vi "总氮总磷质控流程.vi"(0 "队列输入TP":refnum<queue>, 1 "队列输入TN":refnum<queue>, 5 "总氮量程切换":enum32{"H", "L", "AUTO"}(ring)=enum."AUTO", 7 "总磷量程切换":enum32{"H", "L", "AUTO"}(ring)=enum."AUTO", 9 "总磷":bool, 11 "总氮":bool) -> (4 "布尔":bool, 6 "总磷中断报警":bool, 8 "总氮中断报警":bool)   [LabVIEW 2016, in "质控单元.lvlib"]
panel:
  out "总磷":bool
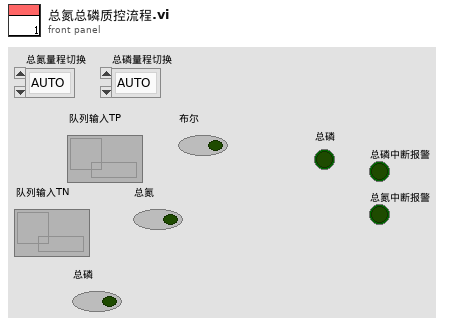
[diagram p1: front panel]
types:
  T1 = enum16{"待机", "启动氨氮水样", "氨氮测量中", "启动氨氮加标", "启动氨氮加标回收", "氨氮加标回收测量中", "启动总氮水样", "总氮测量中", "启动总氮加标", "启动总氮加标回收", "总氮加标回收测量中", "启动总磷水样", "总磷水样测量中", "启动总磷加标", "启动总磷加标回收", "总磷加标回收测量中", "结束"}
  T2 = cluster{"时间标识":timestamp, "设备":string, "日志信息":string}
  T3 = cluster{"站号":u16, "量程切换":enum32{"H", "L", "AUTO"}, "控制命令":enum16{"启动测量", "标样核查", "零点核查", "跨度核查", "空白测试", "平行样测试", "加标回收", "空白校准", "标样校准", "初始化（清洗）", "停止测试", "仪器重启", "校时", "模式设置", "测量间隔设置"}, "模式设置":enum16{"待机", "连续模式", "周期模式", "定点模式", "受控模式", "手动模式"}, "测量间隔":u16}
  T4 = cluster{"系统时间":timestamp, "工作状态":enum16{"空闲", "水样测试", "标样核查", "零点核查", "跨度核查", "空白测试", "平行样测试", "加标回收", "空白校准", "标样校准", "初始化（清洗）"}, "测量模式":enum16{"待机", "连续模式", "周期模式", "定点模式", "受控模式", "手动模式"}, "告警代码":enum16{"无告警", "缺试剂告警", "缺水样告警", "缺蒸馏水告警", "缺标液告警", "仪表漏液告警", "标定异常告警", "超量程告警", "加热异常", "低试剂预警", "超上限告警", "超下限告警", "仪表内部其他异常", "滴定异常告警", "电极异常告警", "量程切换告警", "参数设置告警", "PH电极电位异常", "电导率电极异常", "浊度光度异常", "溶解氧电极异常", "溶解氧光强异常", "温度异常告警", "PH异常告警", "溶解氧异常告警", "电导率异常告警", "浊度异常告警", "叶绿素异常告警", "藻密度异常告警", "蓝绿藻异常告警", "ORP异常告警", "氨氮异常告警", "清洁刷异常告警", "SD卡异常告警", "蓝牙异常告警", "Wifi异常告警", "流程异常告警"}, "故障代码":enum16{"无故障", "电机故障", "温度故障", "通讯故障", "滴定故障"}, "日志代码":u16, "软件版本":u16, "F0":sgl, "F1":sgl, "F2":sgl, "F3":sgl, "T":sgl, "H":sgl, "id":u16, "flowid":u16, "量程":u16, "总磷控温温度1":sgl, "营养盐控温温度2":sgl, "ADC":sgl}
  T5 = enum16{"空闲", "水样测试", "标样核查", "零点核查", "跨度核查", "空白测试", "平行样测试", "加标回收", "空白校准", "标样校准", "初始化（清洗）"}
  T6 = cluster{"因子编码":u32, "单位":u16, "标样参考值":sgl, "水样数据时间":timestamp, "水样实测值":sgl, "水样数据标识":string, "标样数据时间":timestamp, "标样实测值":sgl, "标样数据标识":string, "空白数据时间":timestamp, "空白实测值":sgl, "空白数据标识":string, "零点核查数据时间":timestamp, "零点核查实测值":sgl, "零点核查数据标识":string, "跨度核查数据时间":timestamp, "跨度核查实测值":sgl, "跨度核查数据标识":string, "加标回收数据时间":timestamp, "加标回收实测值":sgl, "加标回收数据标识":string, "平行样数据时间":timestamp, "平行样实测值":sgl, "平行样数据标识":string, "F0":sgl, "F1":sgl, "F2":sgl, "F3":sgl, "F4":sgl, "F5":sgl, "F6":sgl, "F7":sgl, "温度":sgl, "湿度":sgl, "X值":sgl}
  T7 = cluster{"量程":dbl, "检出限":dbl, "加标前水样浓度":dbl, "加标后水样浓度":dbl, "加标水杯定容体积":dbl, "加标母液浓度":dbl, "加标体积":dbl, "加标回收率":dbl}
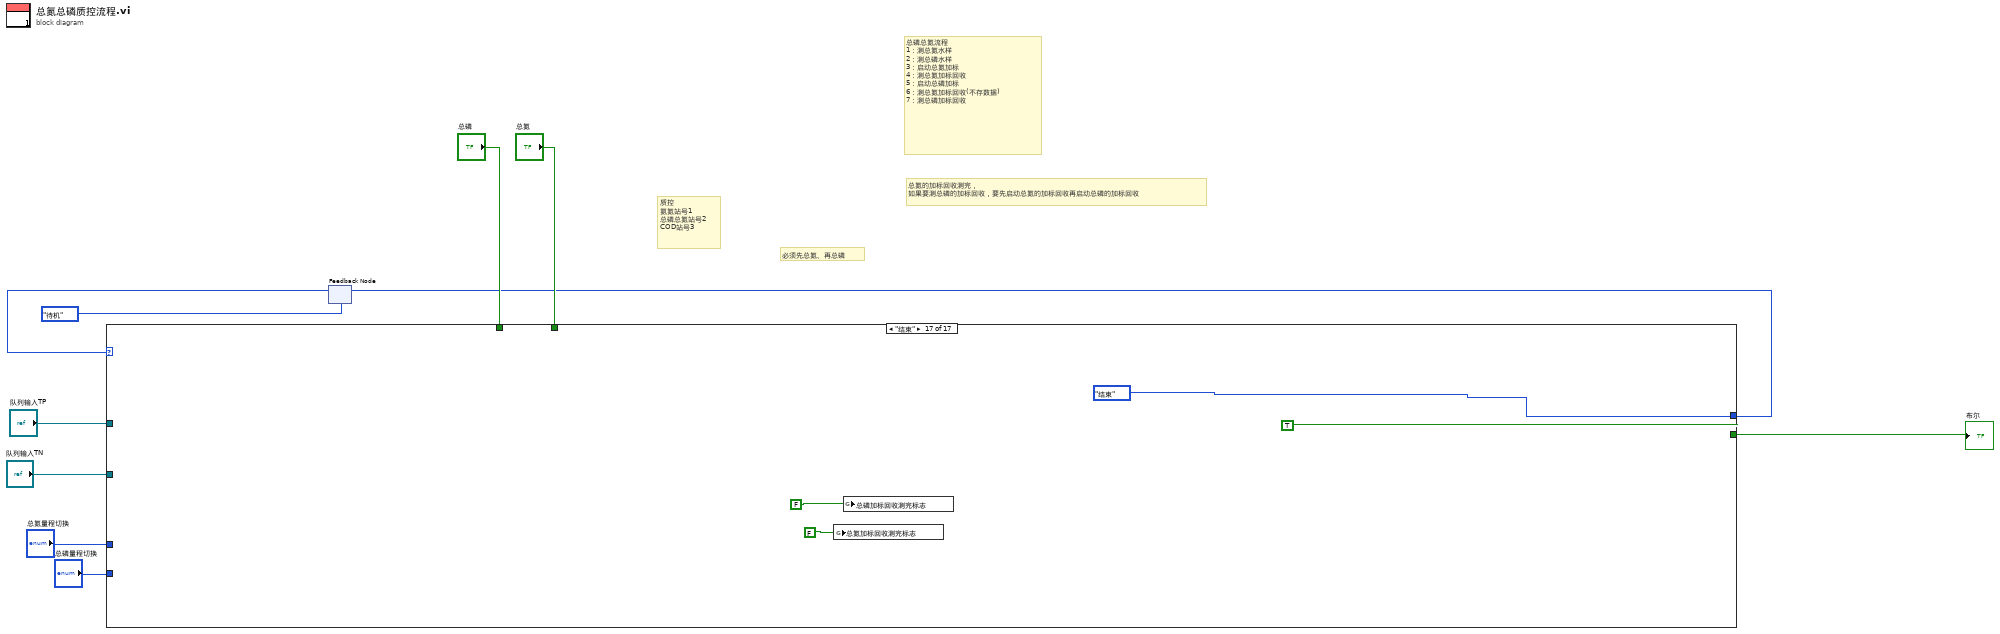
[diagram p0: block diagram]
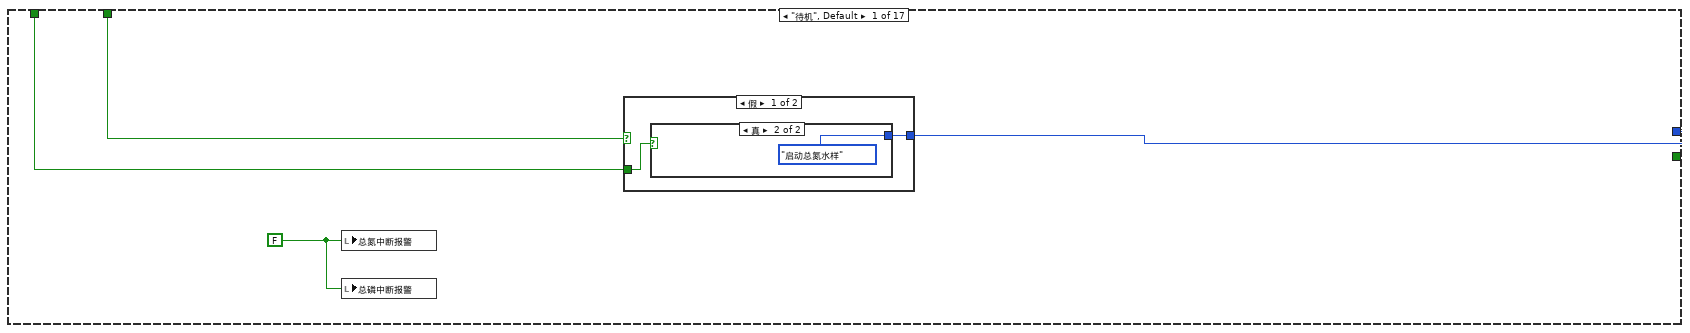
[diagram p2: hidden frame]
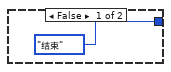
[diagram p3: hidden frame]
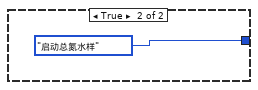
[diagram p4: hidden frame]
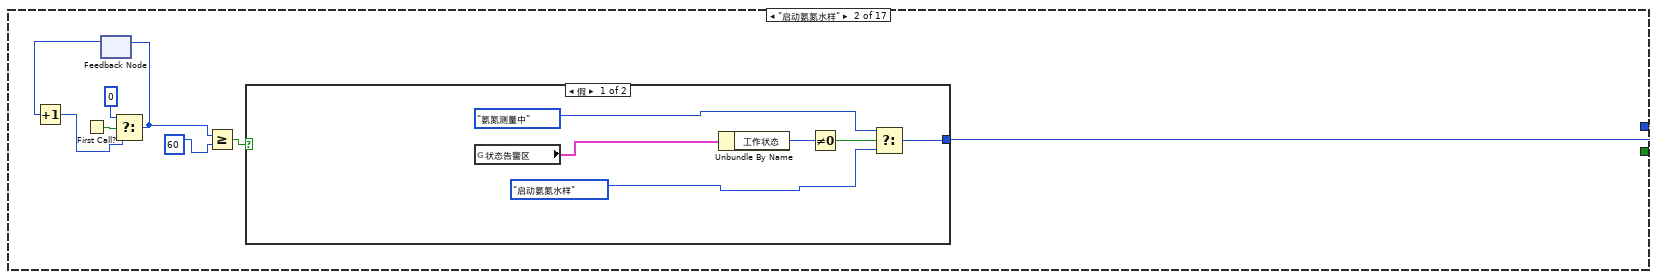
[diagram p5: hidden frame]
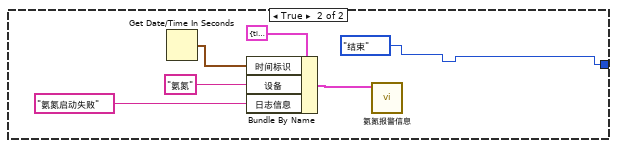
[diagram p6: hidden frame]
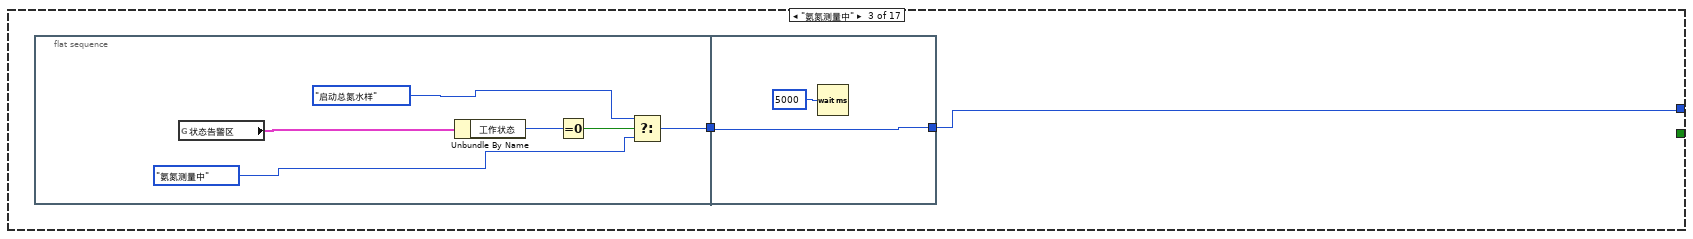
[diagram p7: hidden frame]
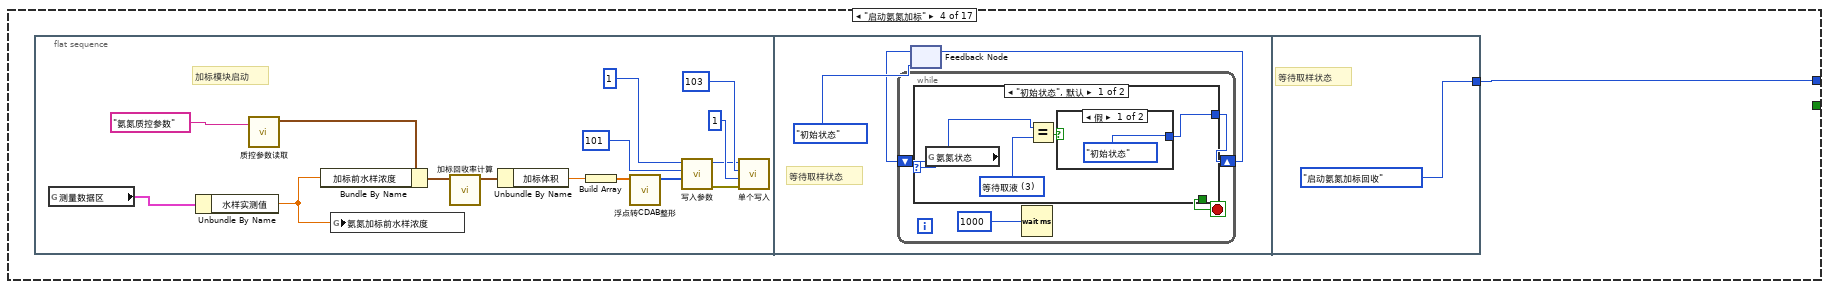
[diagram p8: hidden frame]
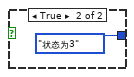
[diagram p9: hidden frame]
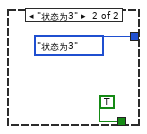
[diagram p10: hidden frame]
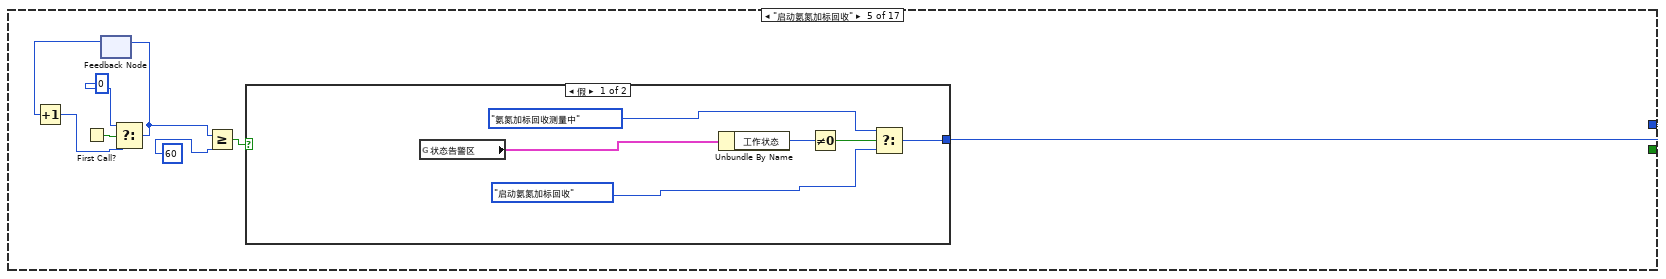
[diagram p11: hidden frame]
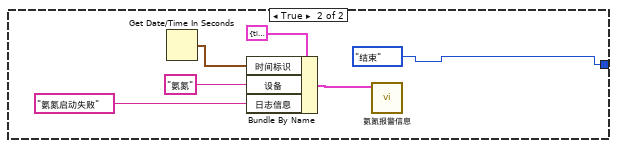
[diagram p12: hidden frame]
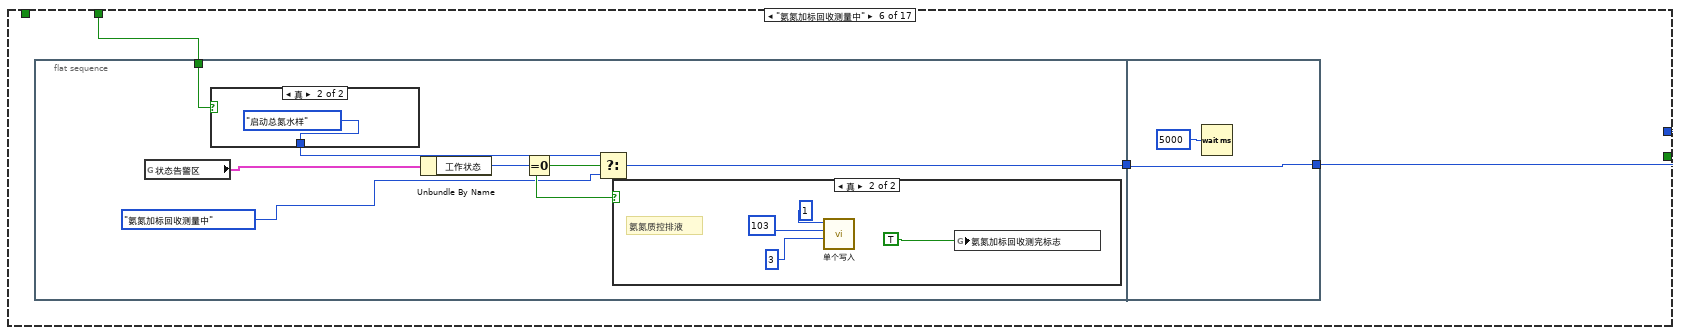
[diagram p13: hidden frame]
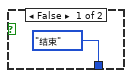
[diagram p14: hidden frame]
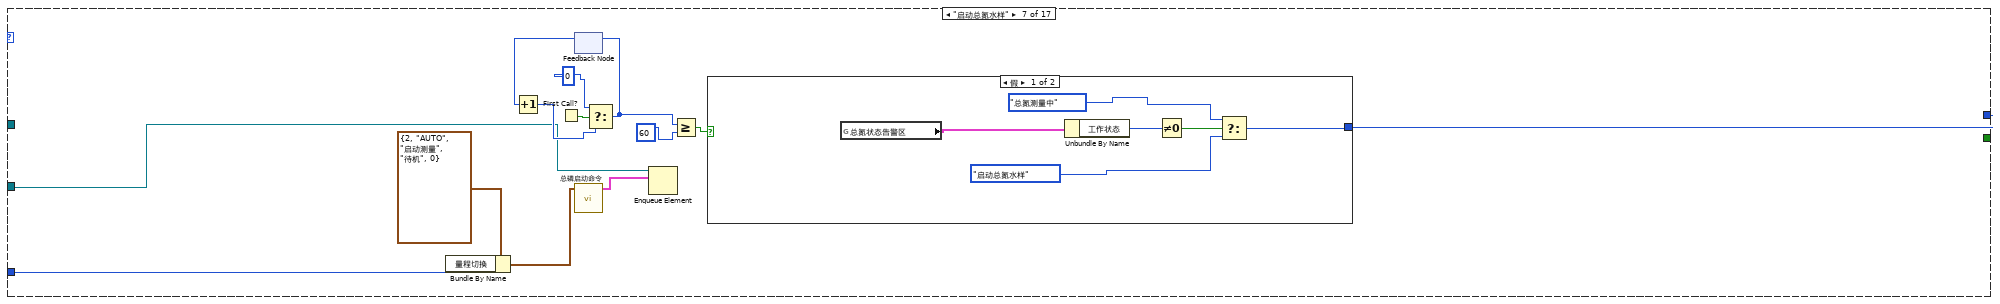
[diagram p16: hidden frame]
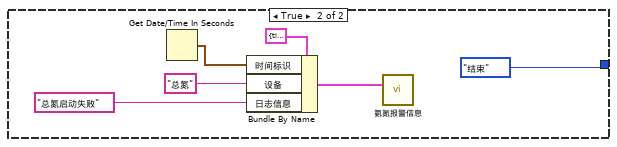
[diagram p17: hidden frame]
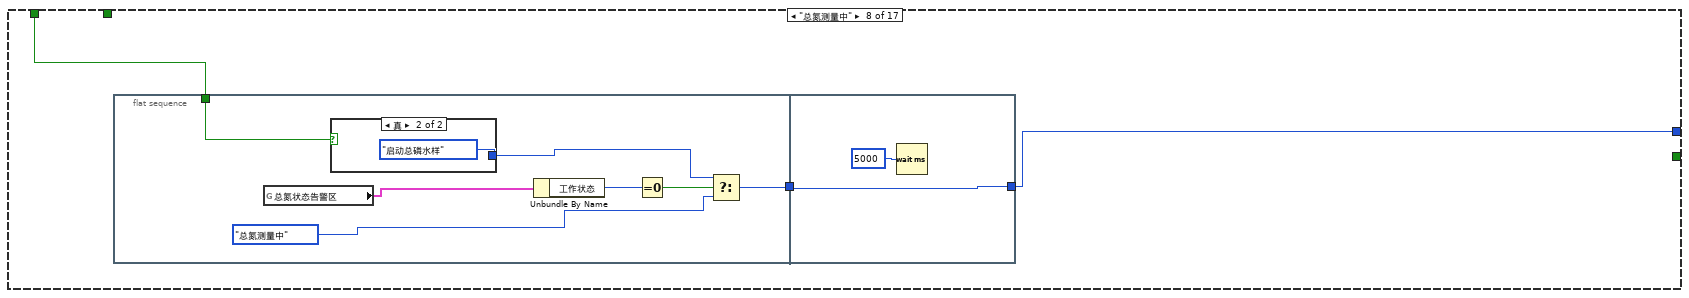
[diagram p18: hidden frame]
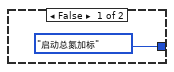
[diagram p19: hidden frame]
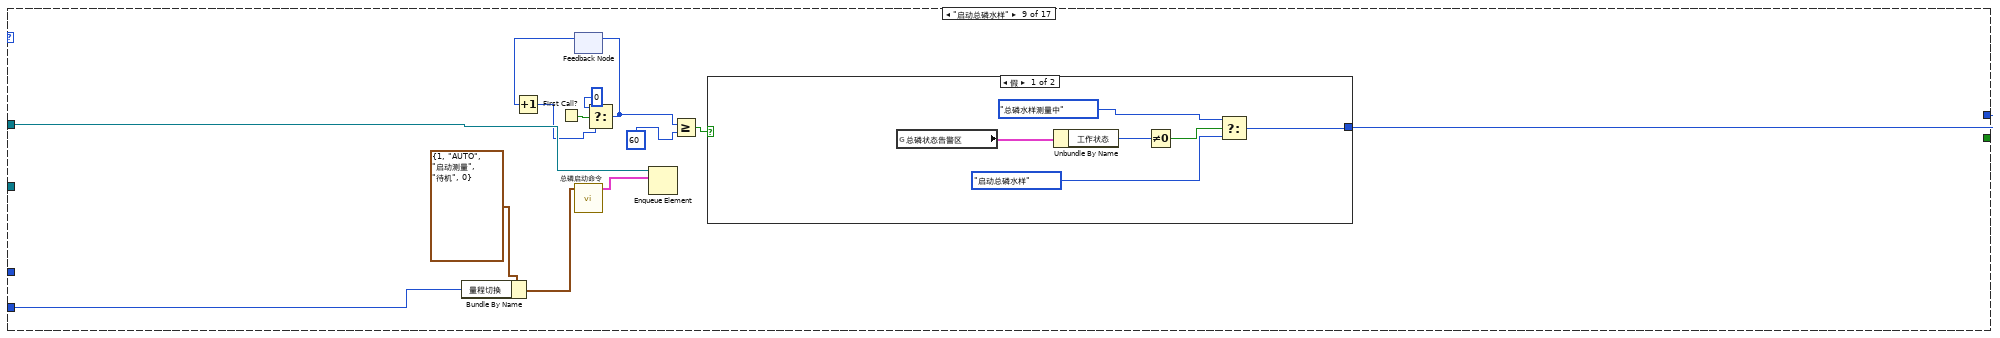
[diagram p20: hidden frame]
diagram:
  # "总磷总氮流程\n1：测总氮水样\n2：测总磷水样\n3：启动总氮加标\n4：测总氮加标回收\n5：启动总磷加标\n6：测总氮加标回收(不存数据)\n7：测总磷加标回收"
  # "总氮的加标回收测完，\n如果要测总磷的加标回收，要先启动总氮的加标回收再启动总磷的加标回收"
  # "质控\n氨氮站号1   \n总磷总氮站号2\nCOD站号3"
  # "必须先总氮、再总磷"
  n1 = feedback #1(T1."待机") -> (w6:T1)
  n2 = case shown="\"结束\"" w6 {
    tunnel: [w14 w27 w41 w50 w81 w101 w131 w145 w169 w185 w197 w238 w260 w288 w331 w353 T1."结束"] -> w4
    tunnel: "队列输入TP" -> [_ _ _ _ _ _ _ _ w170 _ _ _ _ _ w332 _ _]
    tunnel: [_ _ _ _ _ _ _ _ _ _ _ _ _ _ _ _ TRUE] -> w9
    tunnel: "总磷" -> [w13 _ _ _ _ _ _ w144 _ _ _ _ w261 _ _ _ _]
    tunnel: "总氮" -> [w12 _ _ _ _ w102 _ _ _ w183 _ _ w259 _ _ _ _]
    tunnel: "总氮量程切换" -> [_ _ _ _ _ _ w120 _ _ _ _ w235 _ _ _ _ _]
    tunnel: "总磷量程切换" -> [_ _ _ _ _ _ _ _ w158 _ _ _ _ _ w327 _ _]
    tunnel: "队列输入TN" -> [_ _ _ _ _ _ w119 _ _ _ _ w234 _ _ _ _ _]
    frame "待机", Default {
      w11 = FALSE ("总氮中断报警")
      n3 = local write "总氮中断报警"(w11) -> ()
      n4 = local write "总磷中断报警"(w11) -> ()
      n5 = case shown="假" w12 {
        tunnel: w13 -> [w15 _]
        tunnel: [w16 T1."启动总氮水样"] -> w14
        frame False {
          n6 = case shown="真" w15 {
            tunnel: [T1."结束" T1."启动总氮水样"] -> w16
            frame False {
            }
            frame True {
            }
          }
        }
        frame True {
        }
      }
    }
    frame "启动氨氮水样" {
      n7 = First Call?() -> (First Call?: T/F=w25:bool)
      n8 = feedback #2() -> (w24:i32)  [unwired: 1 in]
      n9 = Increment(x=w24) -> (x+1=w23:i32)
      n10 = Select(t=0, s=w25, f=w23) -> (s? t:f=w22:i32)
      n11 = feedback-in #2(w22) -> ()
      n12 = Greater Or Equal?(x=w22, y=60) -> (x >= y?=w20:bool)
      n13 = case shown="假" w20 {
        tunnel: [w31 T1."结束"] -> w27
        frame False {
          n14 = global read "VAR氨氮全局变量.vi" "状态告警区"() -> (w28:T4)
          n15 = Unbundle By Name(w28) -> ("工作状态"=w33:T5)
          n16 = Not Equal To 0?(x=w33) -> (x != 0?=w32:bool)
          n17 = Select(t=T1."氨氮测量中", s=w32, f=T1."启动氨氮水样") -> (s? t:f=w31:T1)
        }
        frame True {
          n18 = Get Date/Time In Seconds() -> (seconds since 1Jan1904=w39:timestamp)
          n19 = Bundle By Name(cluster=T2 {"时间标识"=timestamp(0 s since 1904-01-01), "设备"="", "日志信息"=""} ("data in"), "时间标识"=w39, "设备"="氨氮", "日志信息"="氨氮启动失败") -> (w35:T2)
          n20 = call "氨氮报警信息.vi"("data in"=w35) -> ()  [unwired: 10 in, 1 out]
        }
      }
    }
    frame "氨氮测量中" {
      n21 = flat-sequence {
        tunnel: [w46] -> w40
        tunnel: [w49] -> w41
        tunnel: w40 -> [w49]
        frame #0 {
          n22 = global read "VAR氨氮全局变量.vi" "状态告警区"() -> (w42:T4)
          n23 = Unbundle By Name(w42) -> ("工作状态"=w47:T5)
          n24 = Equal To 0?(x=w47) -> (x = 0?=w45:bool)
          n25 = Select(t=T1."启动总氮水样", s=w45, f=T1."氨氮测量中") -> (s? t:f=w46:T1)
        }
        frame #1 {
          n26 = Wait (ms)(milliseconds to wait=u32 5000 ("等待时间（毫秒）")) -> ()  [unwired: 1 out]
        }
      }
    }
    frame "启动氨氮加标" {
      n27 = flat-sequence {
        tunnel: [T1."启动氨氮加标回收"] -> w50
        frame #0 {
          w54 = u16 1 ("value")
          # "加标模块启动"
          n28 = global read "VAR氨氮全局变量.vi" "测量数据区"() -> (w51:T6)
          n29 = Unbundle By Name(w51) -> ("水样实测值"=w52:sgl)
          n30 = call "质控参数读取.vi"("section"="氨氮质控参数") -> ("参数"=w62:T7)  [unwired: 9 in, 1 out]
          n31 = Bundle By Name(cluster=w62, "加标前水样浓度"=w52) -> (w63:T7)
          n32 = global write "水样浓度全局.vi" "氨氮加标前水样浓度"(w52) -> ()
          n33 = call "加标回收率计算.vi"("参数"=w63) -> ("参数 out"=w61:T7)  [unwired: 10 in]
          n34 = Unbundle By Name(w61) -> ("加标体积"=w53:dbl)
          n35 = Build Array(w53) -> (w60:dbl[])
          n36 = call "浮点转CDAB整形.vi"("浮点数"=w60) -> ("CDAB整形输出"=w55:u16[])  [unwired: 10 in]
          n37 = call "写入参数.vi"("values"=w55, "starting address"=u16 101, "Slave ID"=w54) -> ("error out"=w59:errorcluster)  [unwired: 8 in]
          n38 = call "单个写入.vi"("Error in"=w59, "value"=u16 1, "address"=u16 103, "Slave ID"=w54) -> ()  [unwired: 7 in, 1 out]
        }
        frame #1 {
          # "等待取样状态"
          n39 = feedback #3(enum16{"初始状态", "状态为3"}."初始状态") -> (w66:enum16{"初始状态", "状态为3"})
          n40 = while {
            shift-right: [w70] -> w65
            shift-left: w66 -> [w71]
            stop <- w69 stop-if-true
            n41 = case shown="\"初始状态\", 默认" w71 {
              tunnel: [w73 enum16{"初始状态", "状态为3"}."状态为3"] -> w70
              tunnel: [_ TRUE] -> w69
              frame "初始状态", Default {
                w72 = u16 3 items=["待机", "润洗", "进样", "等待取液", "排液"] ("氨氮状态")
                n42 = global read "氨氮加标回收状态全局变量.vi" "氨氮状态"() -> (w75:u16)
                n43 = Equal?(x=w75, y=w72) -> (x = y?=w74:bool)
                n44 = case shown="假" w74 {
                  tunnel: [enum16{"初始状态", "状态为3"}."初始状态" enum16{"初始状态", "状态为3"}."状态为3"] -> w73
                  frame False {
                  }
                  frame True {
                  }
                }
              }
              frame "状态为3" {
              }
            }
            n45 = Wait (ms)(milliseconds to wait=u32 1000 ("等待时间（毫秒）")) -> ()  [unwired: 1 out]
          }
          n46 = feedback-in #3(w65) -> ()
        }
        frame #2 {
          # "等待取样状态"
        }
      }
    }
    frame "启动氨氮加标回收" {
      n47 = First Call?() -> (First Call?: T/F=w87:bool)
      n48 = feedback #4() -> (w86:i32)  [unwired: 1 in]
      n49 = Increment(x=w86) -> (x+1=w85:i32)
      n50 = Select(t=0, s=w87, f=w85) -> (s? t:f=w84:i32)
      n51 = feedback-in #4(w84) -> ()
      n52 = Greater Or Equal?(x=w84, y=60) -> (x >= y?=w82:bool)
      n53 = case shown="假" w82 {
        tunnel: [w92 T1."结束"] -> w81
        frame False {
          n54 = global read "VAR氨氮全局变量.vi" "状态告警区"() -> (w89:T4)
          n55 = Unbundle By Name(w89) -> ("工作状态"=w94:T5)
          n56 = Not Equal To 0?(x=w94) -> (x != 0?=w93:bool)
          n57 = Select(t=T1."氨氮加标回收测量中", s=w93, f=T1."启动氨氮加标回收") -> (s? t:f=w92:T1)
        }
        frame True {
          n58 = Get Date/Time In Seconds() -> (seconds since 1Jan1904=w100:timestamp)
          n59 = Bundle By Name(cluster=T2 {"时间标识"=timestamp(0 s since 1904-01-01), "设备"="", "日志信息"=""} ("data in"), "时间标识"=w100, "设备"="氨氮", "日志信息"="氨氮启动失败") -> (w96:T2)
          n60 = call "氨氮报警信息.vi"("data in"=w96) -> ()  [unwired: 10 in, 1 out]
        }
      }
    }
    frame "氨氮加标回收测量中" {
      n61 = flat-sequence {
        tunnel: [w109] -> w103
        tunnel: w102 -> [w106]
        tunnel: [w118] -> w101
        tunnel: w103 -> [w118]
        frame #0 {
          n62 = global read "VAR氨氮全局变量.vi" "状态告警区"() -> (w104:T4)
          n63 = case shown="真" w106 {
            tunnel: [T1."结束" T1."启动总氮水样"] -> w108
            frame False {
            }
            frame True {
            }
          }
          n64 = Unbundle By Name(w104) -> ("工作状态"=w110:T5)
          n65 = Equal To 0?(x=w110) -> (x = 0?=w107:bool)
          n66 = Select(t=w108, s=w107, f=T1."氨氮加标回收测量中") -> (s? t:f=w109:T1)
          n67 = case shown="真" w107 {
            frame False {
            }
            frame True {
              # "氨氮质控排液"
              n68 = call "单个写入.vi"("value"=u16 3, "address"=u16 103, "Slave ID"=u8 1) -> ()  [unwired: 8 in, 1 out]
              n69 = global write "质控测完标志全局 1.vi" "氨氮加标回收测完标志"(TRUE) -> ()
            }
          }
        }
        frame #1 {
          n70 = Wait (ms)(milliseconds to wait=u32 5000 ("等待时间（毫秒）")) -> ()  [unwired: 1 out]
        }
      }
    }
    frame "启动总氮水样" {
      n71 = Bundle By Name(cluster=T3 {"站号"=2, "量程切换"=enum."AUTO", "控制命令"=enum."启动测量", "模式设置"=enum."待机", "测量间隔"=0} ("参数"), "量程切换"=w120) -> (w121:T3)
      n72 = First Call?() -> (First Call?: T/F=w129:bool)
      n73 = feedback #5() -> (w128:i32)  [unwired: 1 in]
      n74 = Increment(x=w128) -> (x+1=w127:i32)
      n75 = call "总磷启动命令.vi"("参数"=w121) -> ("启动命令"=w123:cluster{"命令":string, "data":variant})  [unwired: 10 in]
      n76 = Select(t=0, s=w129, f=w127) -> (s? t:f=w126:i32)
      n77 = feedback-in #5(w126) -> ()
      n78 = Enqueue Element(queue=w119, element=w123) -> ()  [unwired: 2 in, 3 out]
      n79 = Greater Or Equal?(x=w126, y=60) -> (x >= y?=w124:bool)
      n80 = case shown="假" w124 {
        tunnel: [w135 T1."结束"] -> w131
        frame False {
          n81 = global read "VAR总氮全局变量.vi" "总氮状态告警区"() -> (w132:T4)
          n82 = Unbundle By Name(w132) -> ("工作状态"=w136:T5)
          n83 = Not Equal To 0?(x=w136) -> (x != 0?=w137:bool)
          n84 = Select(t=T1."总氮测量中", s=w137, f=T1."启动总氮水样") -> (s? t:f=w135:T1)
        }
        frame True {
          n85 = Get Date/Time In Seconds() -> (seconds since 1Jan1904=w143:timestamp)
          n86 = Bundle By Name(cluster=T2 {"时间标识"=timestamp(0 s since 1904-01-01), "设备"="", "日志信息"=""} ("data in"), "时间标识"=w143, "设备"="总氮", "日志信息"="总氮启动失败") -> (w139:T2)
          n87 = call "氨氮报警信息.vi"("data in"=w139) -> ()  [unwired: 10 in, 1 out]
        }
      }
    }
    frame "总氮测量中" {
      n88 = flat-sequence {
        tunnel: [w152] -> w146
        tunnel: w144 -> [w148]
        tunnel: [w157] -> w145
        tunnel: w146 -> [w157]
        frame #0 {
          n89 = global read "VAR总氮全局变量.vi" "总氮状态告警区"() -> (w147:T4)
          n90 = case shown="真" w148 {
            tunnel: [T1."启动总氮加标" T1."启动总磷水样"] -> w150
            frame False {
            }
            frame True {
            }
          }
          n91 = Unbundle By Name(w147) -> ("工作状态"=w153:T5)
          n92 = Equal To 0?(x=w153) -> (x = 0?=w151:bool)
          n93 = Select(t=w150, s=w151, f=T1."总氮测量中") -> (s? t:f=w152:T1)
        }
        frame #1 {
          n94 = Wait (ms)(milliseconds to wait=u32 5000 ("等待时间（毫秒）")) -> ()  [unwired: 1 out]
        }
      }
    }
    frame "启动总磷水样" {
      n95 = Bundle By Name(cluster=T3 {"站号"=1, "量程切换"=enum."AUTO", "控制命令"=enum."启动测量", "模式设置"=enum."待机", "测量间隔"=0} ("参数"), "量程切换"=w158) -> (w159:T3)
      n96 = First Call?() -> (First Call?: T/F=w167:bool)
      n97 = feedback #6() -> (w166:i32)  [unwired: 1 in]
      n98 = Increment(x=w166) -> (x+1=w165:i32)
      n99 = call "总磷启动命令.vi"("参数"=w159) -> ("启动命令"=w161:cluster{"命令":string, "data":variant})  [unwired: 10 in]
      n100 = Select(t=0, s=w167, f=w165) -> (s? t:f=w164:i32)
      n101 = feedback-in #6(w164) -> ()
      n102 = Enqueue Element(queue=w170, element=w161) -> ()  [unwired: 2 in, 3 out]
      n103 = Greater Or Equal?(x=w164, y=60) -> (x >= y?=w162:bool)
      n104 = case shown="假" w162 {
        tunnel: [w173 T1."结束"] -> w169
        frame False {
          n105 = global read "VAR总磷全局变量.vi" "总磷状态告警区"() -> (w174:T4)
          n106 = Unbundle By Name(w174) -> ("工作状态"=w175:T5)
          n107 = Not Equal To 0?(x=w175) -> (x != 0?=w176:bool)
          n108 = Select(t=T1."总磷水样测量中", s=w176, f=T1."启动总磷水样") -> (s? t:f=w173:T1)
        }
        frame True {
          n109 = Get Date/Time In Seconds() -> (seconds since 1Jan1904=w182:timestamp)
          n110 = Bundle By Name(cluster=T2 {"时间标识"=timestamp(0 s since 1904-01-01), "设备"="", "日志信息"=""} ("data in"), "时间标识"=w182, "设备"="总磷", "日志信息"="总磷启动失败") -> (w178:T2)
          n111 = call "氨氮报警信息.vi"("data in"=w178) -> ()  [unwired: 10 in, 1 out]
        }
      }
    }
    frame "总磷水样测量中" {
      n112 = flat-sequence {
        tunnel: [w190] -> w184
        tunnel: w183 -> [w187]
        tunnel: [w196] -> w185
        tunnel: w184 -> [w196]
        frame #0 {
          n113 = case shown="真" w187 {
            tunnel: [T1."启动总磷加标" T1."启动总氮加标"] -> w188
            frame False {
            }
            frame True {
            }
          }
          n114 = global read "VAR总磷全局变量.vi" "总磷状态告警区"() -> (w191:T4)
          n115 = Unbundle By Name(w191) -> ("工作状态"=w192:T5)
          n116 = Equal To 0?(x=w192) -> (x = 0?=w189:bool)
          n117 = Select(t=w188, s=w189, f=T1."总磷水样测量中") -> (s? t:f=w190:T1)
        }
        frame #1 {
          n118 = Wait (ms)(milliseconds to wait=u32 7000 ("等待时间（毫秒）")) -> ()  [unwired: 1 out]
        }
      }
    }
    frame "启动总氮加标" {
      n119 = flat-sequence {
        tunnel: [w231] -> w197
        frame #0 {
          w199 = u16 2 ("value")
          # "加标模块启动"
          n120 = global read "VAR总氮全局变量.vi" "总氮测量数据区"() -> (w198:T6)
          n121 = Unbundle By Name(w198) -> ("水样实测值"=w200:sgl)
          n122 = global write "水样浓度全局.vi" "总氮加标前水样浓度"(w200) -> ()
          n123 = call "质控参数读取.vi"("section"="总氮质控参数") -> ("参数"=w202:T7)  [unwired: 9 in, 1 out]
          n124 = Bundle By Name(cluster=w202, "加标前水样浓度"=w200) -> (w211:T7)
          n125 = Wait (ms)(milliseconds to wait=u32 800 ("等待时间（毫秒）")) -> ()  [unwired: 1 out]
          n126 = call "加标回收率计算.vi"("参数"=w211) -> ("参数 out"=w210:T7)  [unwired: 10 in]
          n127 = Unbundle By Name(w210) -> ("加标体积"=w203:dbl)
          n128 = Build Array(w203) -> (w209:dbl[])
          n129 = call "浮点转CDAB整形.vi"("浮点数"=w209) -> ("CDAB整形输出"=w204:u16[])  [unwired: 10 in]
          n130 = call "写入参数.vi"("values"=w204, "starting address"=u16 101, "Slave ID"=w199) -> ("error out"=w208:errorcluster)  [unwired: 8 in]
          n131 = call "单个写入.vi"("Error in"=w208, "value"=u16 1, "address"=u16 103, "Slave ID"=w199) -> ()  [unwired: 7 in, 1 out]
        }
        frame #1 {
          n132 = Wait (ms)(milliseconds to wait=u32 10000 ("等待时间（毫秒）")) -> ()  [unwired: 1 out]
        }
        frame #2 {
          # "等待取样状态"
          n133 = feedback #7(enum16{"初始状态", "状态为3"}."初始状态") -> (w215:enum16{"初始状态", "状态为3"})
          n134 = while {
            shift-right: [w219] -> w214
            shift-left: w215 -> [w220]
            stop <- w218 stop-if-true
            n135 = case shown="\"初始状态\", 默认" w220 {
              tunnel: [w222 enum16{"初始状态", "状态为3"}."状态为3"] -> w219
              tunnel: [_ TRUE] -> w218
              frame "初始状态", Default {
                n136 = global read "氨氮加标回收状态全局变量.vi" "总氮状态"() -> (w221:u16)
                n137 = case shown="3" w221 {
                  tunnel: [enum16{"初始状态", "状态为3"}."状态为3" enum16{"初始状态", "状态为3"}."初始状态" enum16{"初始状态", "状态为3"}."状态为3"] -> w222
                  frame 0 {
                    "总氮中断报警" <- TRUE ("总氮中断报警")
                  }
                  frame 1, Default {
                  }
                  frame 3 {
                    n138 = local write "总氮中断报警"(FALSE ("总氮中断报警")) -> ()
                  }
                }
              }
              frame "状态为3" {
              }
            }
            n139 = Wait (ms)(milliseconds to wait=u32 1000 ("等待时间（毫秒）")) -> ()  [unwired: 1 out]
          }
          n140 = feedback-in #7(w214) -> ()
        }
        frame #3 {
          # "等待取样状态"
          n141 = local read "总氮中断报警"() -> (w230:bool)
          n142 = case shown="假" w230 {
            tunnel: [T1."启动总氮加标回收" T1."结束"] -> w231
            frame False {
            }
            frame True {
            }
          }
        }
      }
    }
    frame "启动总氮加标回收" {
      n143 = Bundle By Name(cluster=T3 {"站号"=2, "量程切换"=enum."AUTO", "控制命令"=enum."加标回收", "模式设置"=enum."待机", "测量间隔"=0} ("参数"), "量程切换"=w235) -> (w236:T3)
      n144 = First Call?() -> (First Call?: T/F=w245:bool)
      n145 = call "总磷启动命令.vi"("参数"=w236) -> ("启动命令"=w239:cluster{"命令":string, "data":variant})  [unwired: 10 in]
      n146 = feedback #8() -> (w244:i32)  [unwired: 1 in]
      n147 = Increment(x=w244) -> (x+1=w243:i32)
      n148 = Select(t=0, s=w245, f=w243) -> (s? t:f=w242:i32)
      n149 = feedback-in #8(w242) -> ()
      n150 = Enqueue Element(queue=w234, element=w239) -> ()  [unwired: 2 in, 3 out]
      n151 = Greater Or Equal?(x=w242, y=60) -> (x >= y?=w240:bool)
      n152 = case shown="假" w240 {
        tunnel: [w250 T1."结束"] -> w238
        frame False {
          n153 = global read "VAR总氮全局变量.vi" "总氮状态告警区"() -> (w247:T4)
          n154 = Unbundle By Name(w247) -> ("工作状态"=w252:T5)
          n155 = Not Equal To 0?(x=w252) -> (x != 0?=w251:bool)
          n156 = Select(t=T1."总氮加标回收测量中", s=w251, f=T1."启动总氮加标回收") -> (s? t:f=w250:T1)
        }
        frame True {
          n157 = Get Date/Time In Seconds() -> (seconds since 1Jan1904=w258:timestamp)
          n158 = Bundle By Name(cluster=T2 {"时间标识"=timestamp(0 s since 1904-01-01), "设备"="", "日志信息"=""} ("data in"), "时间标识"=w258, "设备"="总氮", "日志信息"="总氮启动失败") -> (w254:T2)
          n159 = call "氨氮报警信息.vi"("data in"=w254) -> ()  [unwired: 10 in, 1 out]
        }
      }
    }
    frame "总氮加标回收测量中" {
      n160 = flat-sequence {
        tunnel: [w272] -> w262
        tunnel: w261 -> [w269]
        tunnel: w259 -> [w265]
        tunnel: [w287] -> w260
        tunnel: w262 -> [w287]
        frame #0 {
          n161 = case shown="真" w269 {
            tunnel: [T1."结束" w276] -> w271
            tunnel: w265 -> [_ w275]
            frame False {
            }
            frame True {
              n162 = case shown="真" w275 {
                tunnel: [T1."启动总磷加标回收" w279] -> w276
                frame False {
                }
                frame True {
                  n163 = local read "总磷"() -> (w278:bool)
                  n164 = case shown="真" w278 {
                    tunnel: [T1."启动总磷加标" T1."启动总磷加标回收"] -> w279
                    frame False {
                    }
                    frame True {
                    }
                  }
                }
              }
            }
          }
          n165 = global read "VAR总氮全局变量.vi" "总氮状态告警区"() -> (w263:T4)
          n166 = Unbundle By Name(w263) -> ("工作状态"=w273:T5)
          n167 = local read "总磷"() -> (w267:bool)
          n168 = Equal To 0?(x=w273) -> (x = 0?=w270:bool)
          n169 = Not(x=w267) -> (.not. x?=w266:bool)
          n170 = And(x=w270, y=w266) -> (x .and. y?=w264:bool)
          n171 = Select(t=w271, s=w270, f=T1."总氮加标回收测量中") -> (s? t:f=w272:T1)
          n172 = case shown="真" w264 {
            frame False {
            }
            frame True {
              # "总氮质控排液"
              n173 = call "单个写入.vi"("value"=u16 3, "address"=u16 103, "Slave ID"=u8 2) -> ()  [unwired: 8 in, 1 out]
              n174 = global write "质控测完标志全局 1.vi" "总氮加标回收测完标志"(TRUE) -> ()
            }
          }
        }
        frame #1 {
          n175 = Wait (ms)(milliseconds to wait=u32 7000 ("等待时间（毫秒）")) -> ()  [unwired: 1 out]
        }
      }
    }
    frame "启动总磷加标" {
      n176 = flat-sequence {
        tunnel: [w324] -> w288
        frame #0 {
          n177 = Wait (ms)(milliseconds to wait=u32 180000 ("等待时间（毫秒）")) -> ()  [unwired: 1 out]
        }
        frame #1 {
          w295 = u16 2 ("value")
          # "加标模块启动"
          n178 = global read "VAR总磷全局变量.vi" "总磷测量数据区"() -> (w291:T6)
          n179 = Unbundle By Name(w291) -> ("水样实测值"=w290:sgl)
          n180 = call "质控参数读取.vi"("section"="总磷质控参数") -> ("参数"=w293:T7)  [unwired: 9 in, 1 out]
          n181 = Bundle By Name(cluster=w293, "加标前水样浓度"=w290) -> (w303:T7)
          n182 = global write "水样浓度全局.vi" "总磷加标前水样浓度"(w290) -> ()
          n183 = Wait (ms)(milliseconds to wait=u32 800 ("等待时间（毫秒）")) -> ()  [unwired: 1 out]
          n184 = call "加标回收率计算.vi"("参数"=w303) -> ("参数 out"=w302:T7)  [unwired: 10 in]
          n185 = Unbundle By Name(w302) -> ("加标体积"=w294:dbl)
          n186 = Build Array(w294) -> (w301:dbl[])
          n187 = call "浮点转CDAB整形.vi"("浮点数"=w301) -> ("CDAB整形输出"=w296:u16[])  [unwired: 10 in]
          n188 = call "写入参数.vi"("values"=w296, "starting address"=u16 101, "Slave ID"=w295) -> ("error out"=w300:errorcluster)  [unwired: 8 in]
          n189 = call "单个写入.vi"("Error in"=w300, "value"=u16 1, "address"=u16 103, "Slave ID"=w295) -> ()  [unwired: 7 in, 1 out]
        }
        frame #2 {
          n190 = Wait (ms)(milliseconds to wait=u32 10000 ("等待时间（毫秒）")) -> ()  [unwired: 1 out]
        }
        frame #3 {
          # "等待取样状态"
          n191 = feedback #9(enum16{"初始状态", "状态为3"}."初始状态") -> (w307:enum16{"初始状态", "状态为3"})
          n192 = while {
            shift-right: [w311] -> w306
            shift-left: w307 -> [w312]
            stop <- w310 stop-if-true
            n193 = case shown="\"状态为3\"" w312 {
              tunnel: [w314 enum16{"初始状态", "状态为3"}."状态为3"] -> w311
              tunnel: [_ TRUE] -> w310
              frame "初始状态", Default {
                n194 = global read "氨氮加标回收状态全局变量.vi" "总磷状态"() -> (w313:u16)
                n195 = case shown="0" w313 {
                  tunnel: [enum16{"初始状态", "状态为3"}."状态为3" enum16{"初始状态", "状态为3"}."初始状态" enum16{"初始状态", "状态为3"}."状态为3"] -> w314
                  frame 0 {
                    "总磷中断报警" <- TRUE ("总磷中断报警")
                  }
                  frame 1, Default {
                  }
                  frame 3 {
                    n196 = local write "总磷中断报警"(FALSE ("总磷中断报警")) -> ()
                  }
                }
              }
              frame "状态为3" {
                "总磷" <- TRUE
              }
            }
            n197 = Wait (ms)(milliseconds to wait=u32 1000 ("等待时间（毫秒）")) -> ()  [unwired: 1 out]
          }
          n198 = feedback-in #9(w306) -> ()
        }
        frame #4 {
          n199 = local read "总磷中断报警"() -> (w323:bool)
          n200 = case shown="假" w323 {
            tunnel: [T1."启动总氮加标回收" T1."结束"] -> w324
            frame False {
              # "等待取样状态"
            }
            frame True {
            }
          }
        }
      }
    }
    frame "启动总磷加标回收" {
      n201 = Bundle By Name(cluster=T3 {"站号"=1, "量程切换"=enum."AUTO", "控制命令"=enum."加标回收", "模式设置"=enum."待机", "测量间隔"=0} ("参数"), "量程切换"=w327) -> (w328:T3)
      n202 = First Call?() -> (First Call?: T/F=w339:bool)
      n203 = feedback #10() -> (w338:i32)  [unwired: 1 in]
      n204 = Increment(x=w338) -> (x+1=w337:i32)
      n205 = call "总磷启动命令.vi"("参数"=w328) -> ("启动命令"=w333:cluster{"命令":string, "data":variant})  [unwired: 10 in]
      n206 = Select(t=0, s=w339, f=w337) -> (s? t:f=w336:i32)
      n207 = feedback-in #10(w336) -> ()
      n208 = Enqueue Element(queue=w332, element=w333) -> ()  [unwired: 2 in, 3 out]
      n209 = Greater Or Equal?(x=w336, y=60) -> (x >= y?=w334:bool)
      n210 = case shown="假" w334 {
        tunnel: [w343 T1."结束"] -> w331
        frame False {
          n211 = global read "VAR总磷全局变量.vi" "总磷状态告警区"() -> (w344:T4)
          n212 = Unbundle By Name(w344) -> ("工作状态"=w345:T5)
          n213 = Not Equal To 0?(x=w345) -> (x != 0?=w346:bool)
          n214 = Select(t=T1."总磷加标回收测量中", s=w346, f=T1."启动总磷加标回收") -> (s? t:f=w343:T1)
        }
        frame True {
          n215 = Get Date/Time In Seconds() -> (seconds since 1Jan1904=w352:timestamp)
          n216 = Bundle By Name(cluster=T2 {"时间标识"=timestamp(0 s since 1904-01-01), "设备"="", "日志信息"=""} ("data in"), "时间标识"=w352, "设备"="总磷", "日志信息"="总磷启动失败") -> (w348:T2)
          n217 = call "氨氮报警信息.vi"("data in"=w348) -> ()  [unwired: 10 in, 1 out]
        }
      }
      n218 = local write "总磷"(FALSE ("总磷")) -> ()
    }
    frame "总磷加标回收测量中" {
      n219 = flat-sequence {
        tunnel: [w358] -> w354
        tunnel: [w366] -> w353
        tunnel: w354 -> [w366]
        frame #0 {
          n220 = global read "VAR总磷全局变量.vi" "总磷状态告警区"() -> (w359:T4)
          n221 = Unbundle By Name(w359) -> ("工作状态"=w360:T5)
          n222 = Equal To 0?(x=w360) -> (x = 0?=w357:bool)
          n223 = Select(t=T1."结束", s=w357, f=T1."总磷加标回收测量中") -> (s? t:f=w358:T1)
          n224 = case shown="真" w357 {
            frame False {
            }
            frame True {
              # "总磷质控排液"
              n225 = global write "质控测完标志全局 1.vi" "总磷加标回收测完标志"(TRUE) -> ()
              n226 = call "单个写入.vi"("value"=u16 3, "address"=u16 103, "Slave ID"=u8 2) -> ()  [unwired: 8 in, 1 out]
            }
          }
        }
        frame #1 {
          n227 = Wait (ms)(milliseconds to wait=u32 5000 ("等待时间（毫秒）")) -> ()  [unwired: 1 out]
        }
      }
    }
    frame "结束" {
      n228 = global write "质控测完标志全局 1.vi" "总氮加标回收测完标志"(FALSE) -> ()
      n229 = global write "质控测完标志全局 1.vi" "总磷加标回收测完标志"(FALSE) -> ()
    }
  }
  "布尔" <- w9
  n230 = feedback-in #1(w4) -> ()
